vi "send_trigger.vi"(8 "error in (no error)":errorcluster, 10 "message":T1, 11 "ScanModeTS090821Circular2D in":refnum<class "ScanModeTS090821Circular2D.lvclass">=refnum) -> (0 "error out":errorcluster, 3 "ScanModeTS090821Circular2D out":refnum<class "ScanModeTS090821Circular2D.lvclass">)   [LabVIEW 2010]
uses:
  main/labview_source/type_definitions/classes/GenericScanMode/class_data.vi
  ScanModeTS090821Circular2D_statechart.lvsc/Trigger.ctl
  main/labview_source/type_definitions/classes/GenericScanMode/trigger_enum.ctl
  ScanModeTS090821Circular2D.lvclass
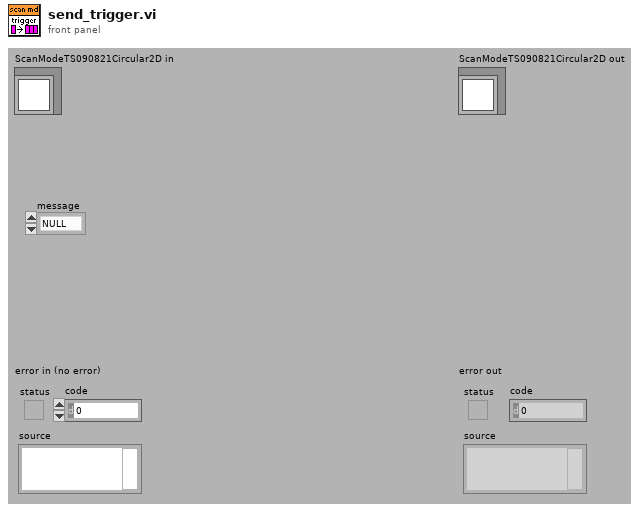
[diagram p1: front panel]
types:
  T1 = typedef "GenericScanMode.lvclass/trigger_enum.ctl" = enum16{"NULL", "initialise", "terminate", "start", "stop", "proceed"}
  T2 = typedef "ScanModeTS090821Circular2D_statechart.lvsc/Trigger.ctl" = enum16{"NULL", "initialise", "terminate", "start", "stop", "update", "sweep finished"}
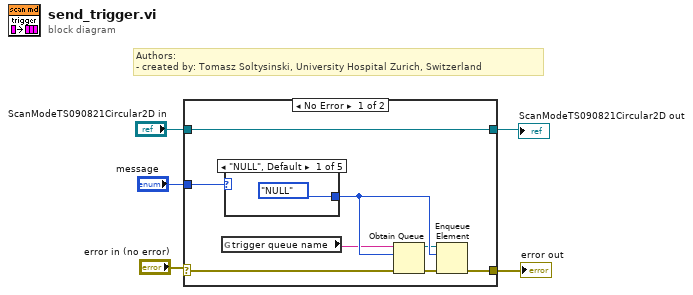
[diagram p0: block diagram]
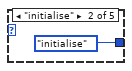
[diagram p2: hidden frame]
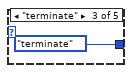
[diagram p3: hidden frame]
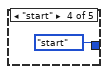
[diagram p4: hidden frame]
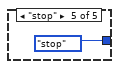
[diagram p5: hidden frame]
diagram:
  # "Authors: \n- created by: Tomasz Soltysinski, University Hospital Zurich, Switzerland"
  n1 = case shown="No Error" "error in (no error)" {
    selector: "error in (no error)" -> [w8 w20]
    tunnel: [w7 w20] -> w2
    tunnel: [w13 w19] -> w1
    tunnel: "ScanModeTS090821Circular2D in" -> [w13 w19]
    tunnel: "message" -> [w12 _]
    frame No Error {
      n2 = global read "class_data.vi" "trigger queue name"() -> (w6:string)
      n3 = case shown="\"NULL\", Default" w12 {
        tunnel: [Trigger."NULL" ("Trigger") Trigger."initialise" ("Trigger") Trigger."terminate" ("Trigger") Trigger."start" ("Trigger") Trigger."stop" ("Trigger")] -> w11
        frame "NULL", Default {
        }
        frame "initialise" {
        }
        frame "terminate" {
        }
        frame "start" {
        }
        frame "stop" {
        }
      }
      n4 = Obtain Queue(name (unnamed)=w6, element data type=w11, error in (no error)=w8) -> (queue out=w10:refnum<queue>, error out=w9:errorcluster)  [unwired: 2 in, 1 out]
      n5 = Enqueue Element(queue=w10, element=w11, error in (no error)=w9) -> (error out=w7:errorcluster)  [unwired: 3 out]
    }
    frame Error {
    }
  }
  "error out" <- w2
  "ScanModeTS090821Circular2D out" <- w1
